vi "RT Main.vi"() -> ()   [LabVIEW 2019]
doc: "The myRIO Custom FPGA Project template acquires button data from the onboard button and displays the button value on a Boolean indicator. The SYS.RDY indicator shows the FPGA status."
uses:
  <vilib>/myRIO/Instrument Drivers/Onboard IO/DIO/typedefs/DIO Reference.ctl
  <vilib>/myRIO/Common/Instrument Driver Framework/Utilities/typedefs/myRIO Generic Hardware Reference.ctl
  <vilib>/myRIO/Common/Instrument Driver Framework/Utilities/typedefs/Hardware Version Enum.ctl
  <vilib>/myRIO/Common/Instrument Driver Framework/Utilities/typedefs/myRIO v1.0 Reference.ctl
  <vilib>/myRIO/Common/Instrument Driver Framework/Utilities/typedefs/Generic FPGA Reference.ctl
  <vilib>/myRIO/Common/Instrument Driver Framework/myRIO v1.0/DIO/typedefs/DIO Channels List.ctl
  <vilib>/myRIO/Common/Instrument Driver Framework/myRIO v1.0/DIO/typedefs/DIO Channels Enum.ctl
  <vilib>/userDefined/High Color/nirio_resource_hc.ctl
  <vilib>/myRIO/Common/Instrument Driver Framework/myRIO v1.0/DIO/vis/myRIO v1.1 Open DIO.vi
  <vilib>/myRIO/Common/Instrument Driver Framework/Utilities/vis/Validate Channels.vi
  <vilib>/myRIO/Common/Instrument Driver Framework/myRIO v1.0/DIO/vis/myRIO v1.0 Reserve DIO.vi
  <vilib>/myRIO/Common/Instrument Driver Framework/myRIO v1.0/Resource Manager/vis/myRIO v1.0 Reserve Channel List.vi
  <vilib>/myRIO/Common/Instrument Driver Framework/myRIO v1.0/DIO/vis/myRIO v1.0 Build MUX Configuration DIO.vi
  <vilib>/myRIO/Common/Instrument Driver Framework/myRIO v1.0/Resource Manager/vis/myRIO v1.0 Reserve Channel.vi
  <vilib>/myRIO/Common/Instrument Driver Framework/myRIO v1.0/Resource Manager/vis/myRIO v1.0 Unreserve Channel.vi
  <vilib>/myRIO/Common/Instrument Driver Framework/myRIO v1.0/Resource Manager/vis/myRIO v1.0 Create Configuration List.vi
  <vilib>/myRIO/Common/Instrument Driver Framework/myRIO v1.0/Resource Manager/vis/myRIO v1.0 Build Mutex Name.vi
  <vilib>/Utility/VariantDataType/GetNumericInfo.vi
  <vilib>/Utility/error.llb/Error Cluster From Error Code.vi
  <vilib>/myRIO/Common/Instrument Driver Framework/myRIO v1.0/myRIO v1.1 Open.vi
  <vilib>/myRIO/Common/Instrument Driver Framework/Utilities/vis/IO Manager.vi
  <vilib>/myRIO/Common/Instrument Driver Framework/Utilities/vis/Configuration Manager.vi
  <vilib>/myRIO/Common/Instrument Driver Framework/myRIO v1.0/Resource Manager/vis/myRIO v1.0 Configure IO.vi
  <vilib>/myRIO/Common/Instrument Driver Framework/myRIO v1.0/myRIO v1.0 Close.vi
  <vilib>/myRIO/Common/Instrument Driver Framework/myRIO v1.0/DIO/vis/myRIO v1.0 Write DIO.vi
  <vilib>/myRIO/Instrument Drivers/Onboard IO/DIO/vis/myRIO DIO Open.xnode
  <vilib>/myRIO/Instrument Drivers/Onboard IO/DIO/DIO.lvlib
panel:
  in  "Channel Names":tag[](array[tag])
  in  "y":i32
  in  "Tick Count(uSec) 2":u32 caption="Tick Count(uSec)"
  in  "Tick Count(uSec)":u32
  out "error out":errorcluster
  in  "error in (no error)":errorcluster
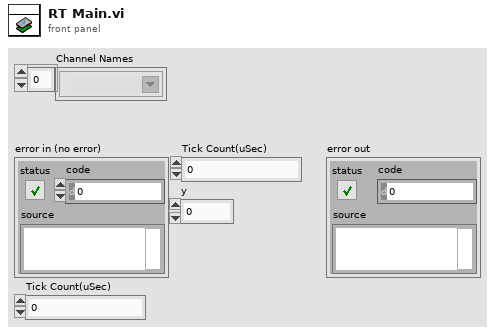
[diagram p1: front panel]
types:
  T1 = typedef "nirio_resource_hc.ctl" = tag
  T2 = typedef "Hardware Version Enum.ctl" = enum16{"Unknown", "myRIO-1900", "myRIO-1950", "roboRIO", "NI ELVIS RIO CM", "ELVIS III"}
  T3 = typedef "DIO.lvlib/DIO Reference.ctl" = cluster{"myRIO Reference":T4, "DIO Channels List":T7}
  T4 = typedef "myRIO Generic Hardware Reference.ctl" = cluster{"myRIO Model":T2, "myRIO Hardware Reference":T5}
  T5 = typedef "myRIO v1.0 Reference.ctl" = cluster{"Generic FPGA Reference":T6, "Allow multiple opens":bool}
  T6 = typedef "Generic FPGA Reference.ctl" = refnum<k20>
  T7 = typedef "DIO Channels List.ctl" = T8[]
  T8 = typedef "DIO Channels Enum.ctl" = enum16{"Not Connected", "C/DIO0", "C/DIO1", "C/DIO2", "C/DIO3", "C/DIO4", "C/DIO5", "C/DIO6", "C/DIO7", "A/DIO0", "A/DIO1", "A/DIO2", "A/DIO3", "A/DIO4", "A/DIO5", "A/DIO6", "A/DIO7", "A/DIO8", "A/DIO9", "A/DIO10", "A/DIO11", "A/DIO12", "A/DIO13", "A/DIO14", "A/DIO15", "A/DIO16", "A/DIO17", "A/DIO18", "A/DIO19", "B/DIO0", "B/DIO1", "B/DIO2", "B/DIO3", "B/DIO4", "B/DIO5", "B/DIO6", "B/DIO7", "B/DIO8", "B/DIO9", "B/DIO10", "B/DIO11", "B/DIO12", "B/DIO13", "B/DIO14", "B/DIO15", "B/DIO16", "B/DIO17", "B/DIO18", "B/DIO19", "LED0", "LED1", "LED2", "LED3", "Button0", "DIO/DIO0", "DIO/DIO1", "DIO/DIO2", "DIO/DIO3", "DIO/DIO4", "DIO/DIO5", "DIO/DIO6", "DIO/DIO7", "DIO/DIO8", "DIO/DIO9", "SPI/CS0", "SPI/CS1", "SPI/CS2", "SPI/CS3", "LED RADIO (Green)", "LED RADIO (Red)", "LED COMM (Green)", "LED COMM (Red)", "LED MODE (Green)", "LED MODE (Red)"}
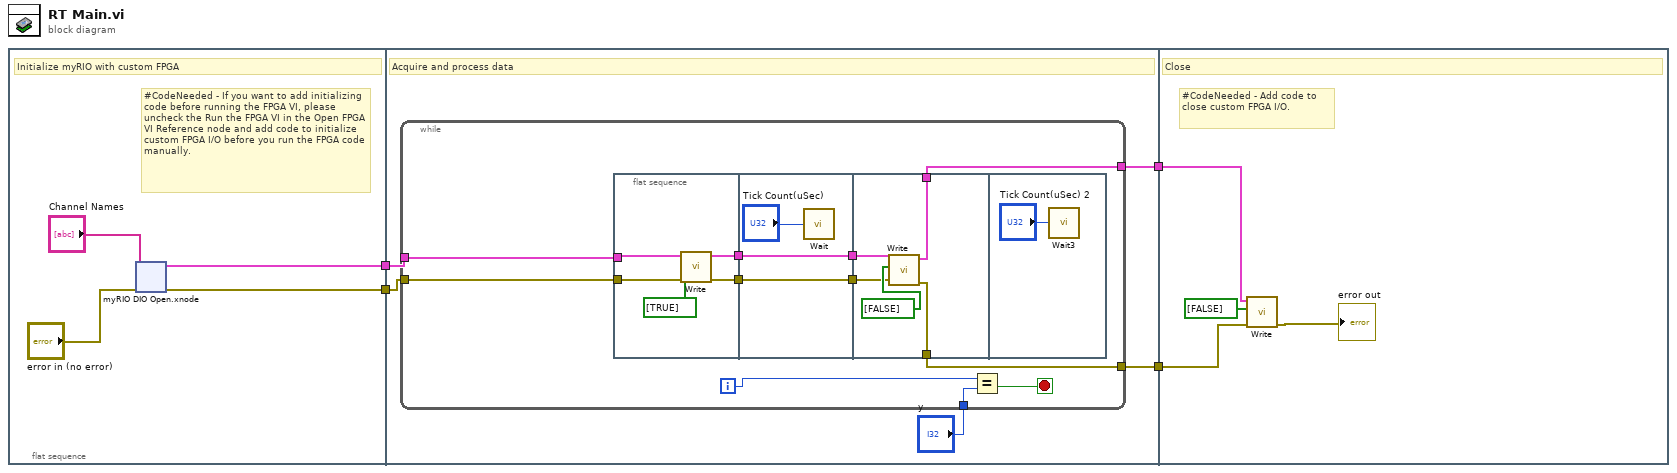
[diagram p0: block diagram]
diagram:
  n1 = flat-sequence {
    tunnel: [w7] -> w4
    tunnel: [w6] -> w3
    tunnel: w4 -> [w28]
    tunnel: w3 -> [w29]
    tunnel: [w27] -> w2
    tunnel: [w25] -> w1
    tunnel: w2 -> [w58]
    tunnel: w1 -> [w56]
    frame #0 {
      # "#CodeNeeded - If you want to add initializing code before running the FPGA VI, please uncheck the Run the FPGA VI in the Open FPGA VI Reference node and add code to initialize custom FPGA I/O before you run the FPGA code manually."
      # "Initialize myRIO with custom FPGA"
      n2 = xnode "myRIO DIO Open.xnode"("error in (no error)"="error in (no error)", "Channel Names"="Channel Names") -> ("error out"=w7:errorcluster, "DIO Ref Out"=w6:T3)  [unwired: 1 in]
    }
    frame #1 {
      # "Acquire and process data"
      n3 = while {
        tunnel: w29 -> [w40]
        tunnel: w28 -> [w37]
        tunnel: [w34] -> w27
        tunnel: "y" -> [w31]
        tunnel: [w30] -> w25
        i -> [w32]
        stop <- w33 stop-if-true
        n4 = flat-sequence {
          tunnel: w40 -> [w45]
          tunnel: [w43] -> w38
          tunnel: w37 -> [w42]
          tunnel: [w41] -> w35
          tunnel: [w47] -> w39
          tunnel: w38 -> [w47]
          tunnel: [w46] -> w36
          tunnel: w35 -> [w46]
          tunnel: w39 -> [w53]
          tunnel: w36 -> [w51]
          tunnel: [w50] -> w34
          tunnel: [w49] -> w30
          frame #0 {
            n5 = call <vilib>:"Write.vi"("error in (no error)"=w42, "Values"=bool[] [TRUE], "DIO Ref In"=w45) -> ("error out"=w41:errorcluster, "DIO Ref Out"=w43:T3)  [unwired: 6 in]
          }
          frame #1 {
            n6 = call "Wait"("Count(uSec)"="Tick Count(uSec)") -> ()  [unwired: 1 out]
          }
          frame #2 {
            n7 = call <vilib>:"Write.vi"("error in (no error)"=w51, "Values"=bool[] [FALSE], "DIO Ref In"=w53) -> ("error out"=w50:errorcluster, "DIO Ref Out"=w49:T3)  [unwired: 6 in]
          }
          frame #3 {
            n8 = call "Wait3"("Count(uSec)"="Tick Count(uSec) 2") -> ()  [unwired: 1 out]
          }
        }
        n9 = Equal?(x=w32, y=w31) -> (x = y?=w33:bool)
      }
    }
    frame #2 {
      # "#CodeNeeded - Add code to close custom FPGA I/O."
      # "Close"
      n10 = call <vilib>:"Write.vi"("error in (no error)"=w58, "Values"=bool[] [FALSE], "DIO Ref In"=w56) -> ("error out"=→"error out":errorcluster)  [unwired: 6 in, 1 out]
    }
  }
